vi "Write Queue Reference.vi"(8 "error in (no error)":errorcluster, 10 "Queue Reference":refnum<queue>[](array[refnum]), 11 "ModuleAdmin in":refnum<class "ModuleAdmin.lvclass">) -> (0 "error out":errorcluster, 3 "ModuleAdmin out":refnum<class "ModuleAdmin.lvclass">)   [LabVIEW 2018, in "ModuleAdmin.lvlib" / "ModuleAdmin.lvclass"]
uses:
  ModuleAdmin.lvclass
  ModuleAdmin.lvclass/ModuleAdmin.ctl
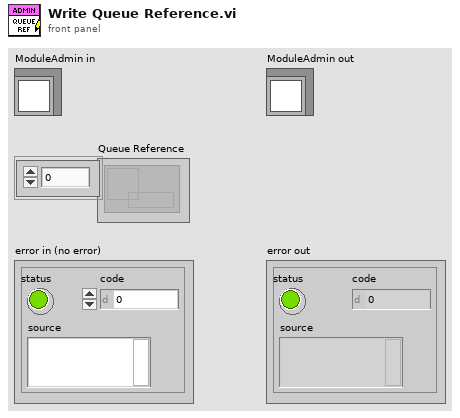
[diagram p1: front panel]
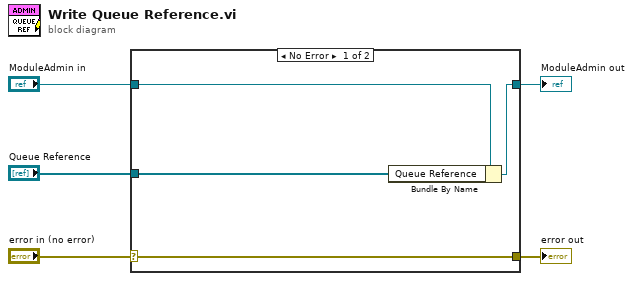
[diagram p0: block diagram]
diagram:
  n1 = case shown="No Error" "error in (no error)" {
    selector: "error in (no error)" -> [w9 w10]
    tunnel: [w9 w10] -> w4
    tunnel: [w7 w11] -> w2
    tunnel: "ModuleAdmin in" -> [w8 w11]
    tunnel: "Queue Reference" -> [w6 _]
    frame No Error {
      n2 = Bundle By Name(cluster=w8, "Queue Reference"=w6) -> (w7:refnum<class "ModuleAdmin.lvclass">)
    }
    frame Error {
    }
  }
  "error out" <- w4
  "ModuleAdmin out" <- w2
